vi "Untitled 2.vi"() -> ()   [LabVIEW 2014]
panel:
  out "Boolean 2":bool
  out "String":string
  in  "password":T1
  # "Siavash Aghajani"
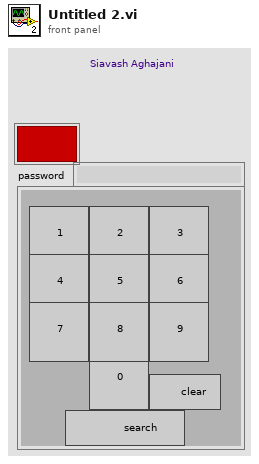
[diagram p1: front panel]
types:
  T1 = cluster{"Blank Button 2":bool, "Blank Button 3":bool, "Blank Button 4":bool, "Blank Button 5":bool, "Blank Button 6":bool, "Blank Button 7":bool, "Blank Button 8":bool, "Blank Button 9":bool, "Blank Button 10":bool, "Blank Button":bool, "Blank Button 11":bool, bool}
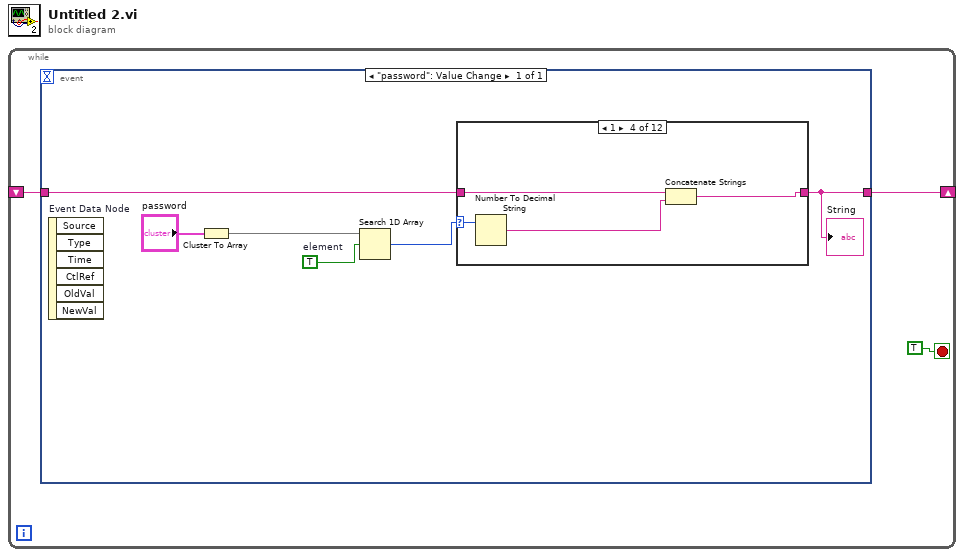
[diagram p0: block diagram]
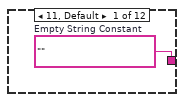
[diagram p2: hidden frame]
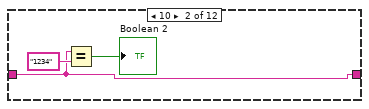
[diagram p3: hidden frame]
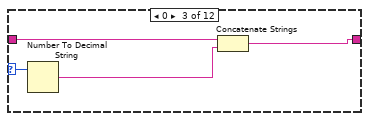
[diagram p4: hidden frame]
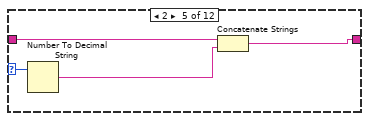
[diagram p5: hidden frame]
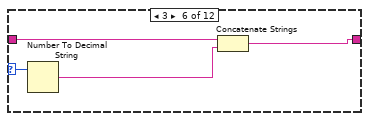
[diagram p6: hidden frame]
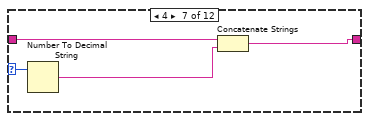
[diagram p7: hidden frame]
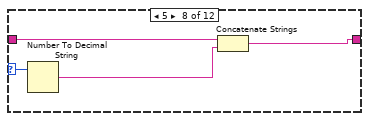
[diagram p8: hidden frame]
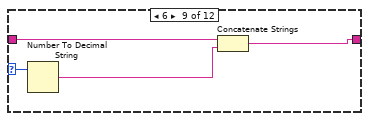
[diagram p9: hidden frame]
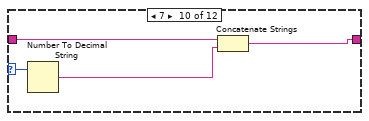
[diagram p10: hidden frame]
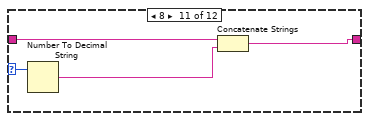
[diagram p11: hidden frame]
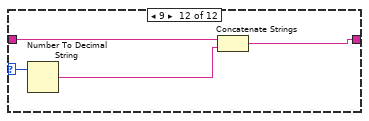
[diagram p12: hidden frame]
diagram:
  n1 = while {
    shift-right: [w1] -> _
    shift-left: _ -> [w2]
    stop <- TRUE stop-if-true
    n2 = event shown="[0] \"password\": Value Change" {
      selector: _ -> [_]
      dyn-events: _ -> [_]
      timeout: _ -> [_]
      tunnel: w2 -> [w6]
      tunnel: [w5] -> w1
      event "password": Value Change {
        w7 = TRUE  # element
        n3 = event-data "Event Data Node"() -> ()  [unwired: 1 in, 6 out]
        n4 = Cluster To Array(cluster="password") -> (array=w9:bool[])
        n5 = Search 1D Array(1D array=w9, element=w7) -> (index of element=w4:i32)  [unwired: 1 in]
        n6 = case shown="1" w4 {
          selector: w4 -> [_ _ w14 w18 w22 w26 w30 w34 w38 w42 w46 w50]
          tunnel: w6 -> [_ w12 w16 w20 w24 w28 w32 w36 w40 w44 w48 w52]
          tunnel: [w10 w12 w15 w19 w23 w27 w31 w35 w39 w43 w47 w51] -> w5
          frame 11, Default {
            w10 = ""  # Empty String Constant
          }
          frame 10 {
            n7 = Equal?(x=w12, y="1234") -> (x = y?=→"Boolean 2":bool)
          }
          frame 0 {
            n8 = Number To Decimal String(number=w14) -> (decimal integer string=w17:string)  [unwired: 1 in]
            n9 = Concatenate Strings "Concatenate Strings"(w16, w17) -> (w15:string)
          }
          frame 1 {
            n10 = Number To Decimal String(number=w18) -> (decimal integer string=w21:string)  [unwired: 1 in]
            n11 = Concatenate Strings "Concatenate Strings"(w20, w21) -> (w19:string)
          }
          frame 2 {
            n12 = Number To Decimal String(number=w22) -> (decimal integer string=w25:string)  [unwired: 1 in]
            n13 = Concatenate Strings "Concatenate Strings"(w24, w25) -> (w23:string)
          }
          frame 3 {
            n14 = Number To Decimal String(number=w26) -> (decimal integer string=w29:string)  [unwired: 1 in]
            n15 = Concatenate Strings "Concatenate Strings"(w28, w29) -> (w27:string)
          }
          frame 4 {
            n16 = Number To Decimal String(number=w30) -> (decimal integer string=w33:string)  [unwired: 1 in]
            n17 = Concatenate Strings "Concatenate Strings"(w32, w33) -> (w31:string)
          }
          frame 5 {
            n18 = Number To Decimal String(number=w34) -> (decimal integer string=w37:string)  [unwired: 1 in]
            n19 = Concatenate Strings "Concatenate Strings"(w36, w37) -> (w35:string)
          }
          frame 6 {
            n20 = Number To Decimal String(number=w38) -> (decimal integer string=w41:string)  [unwired: 1 in]
            n21 = Concatenate Strings "Concatenate Strings"(w40, w41) -> (w39:string)
          }
          frame 7 {
            n22 = Number To Decimal String(number=w42) -> (decimal integer string=w45:string)  [unwired: 1 in]
            n23 = Concatenate Strings "Concatenate Strings"(w44, w45) -> (w43:string)
          }
          frame 8 {
            n24 = Number To Decimal String(number=w46) -> (decimal integer string=w49:string)  [unwired: 1 in]
            n25 = Concatenate Strings "Concatenate Strings"(w48, w49) -> (w47:string)
          }
          frame 9 {
            n26 = Number To Decimal String(number=w50) -> (decimal integer string=w53:string)  [unwired: 1 in]
            n27 = Concatenate Strings "Concatenate Strings"(w52, w53) -> (w51:string)
          }
        }
        "String" <- w5
      }
    }
  }
